vi "GenerateHeaderAndFilename.vi"(0 "Computer":string, 1 "Instrument Information":string, 2 "Test Name":string, 3 "Payload vi Name":string, 4 "Ssid":string="<tba>", 5 "Setup vi Name":string, 6 "Test Parameter File Name":string, 7 "Input Constants Keys":i32[](array[numeric]), 8 "SN":string, 9 "Input Constants Names":string[](array[string]), 10 "BenchId":string, 11 "Input Constants Values":string[](array[string])) -> (15 "Header":string[](array[string]), 18 "Filename Path":path)   [LabVIEW 2018]
uses:
  Test Result File Name Global.vi
  Automated Tests/Tetra WAM/Tetra_Globals.vi
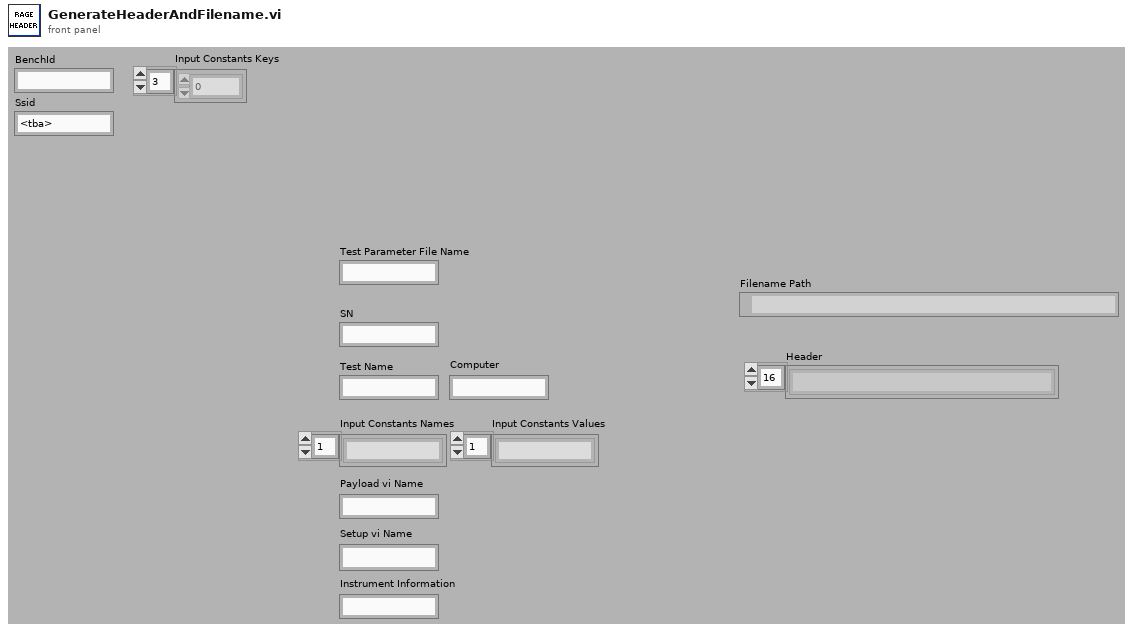
[diagram p1: front panel]
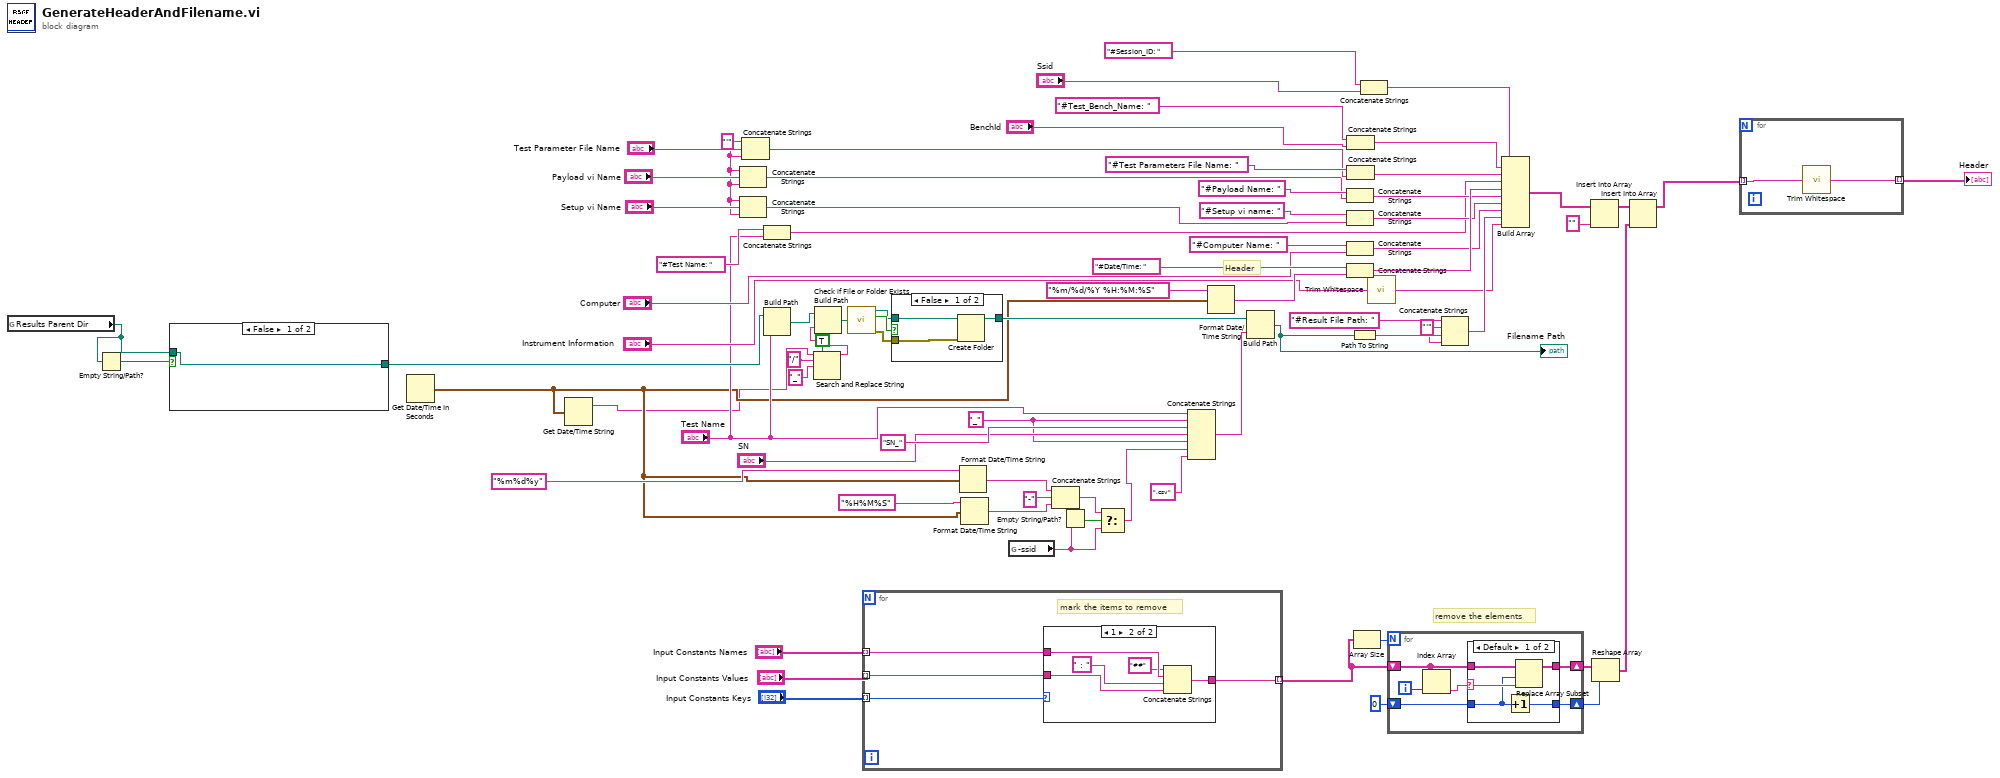
[diagram p0: block diagram]
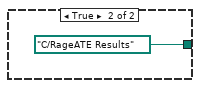
[diagram p3: hidden frame]
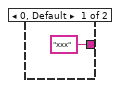
[diagram p5: hidden frame]
diagram:
  w13 = "'" ("string")
  w21 = "'" ("string")
  w36 = "_" ("string")
  # "remove the elements"
  # "Header"
  n1 = global read "Test Result File Name Global.vi" "Results Parent Dir"() -> (w33:path)
  n2 = Empty String/Path?(string/path=w33) -> (empty?=w34:bool)
  n3 = case shown="False" w34 {
    tunnel: [w80 path "C:/RageATE Results" ("base path")] -> w55
    tunnel: w33 -> [w80 _]
    frame False {
    }
    frame True {
    }
  }
  n4 = Get Date/Time In Seconds() -> (seconds since 1Jan1904=w19:timestamp)
  n5 = Get Date/Time String(seconds (now)=w19) -> (date string=w18:string)  [unwired: 2 in, 1 out]
  n6 = Concatenate Strings(w13, "Payload vi Name", w13) -> (w15:string)
  n7 = Concatenate Strings(w13, "Setup vi Name", w13) -> (w14:string)
  n8 = Concatenate Strings(w13, "Test Parameter File Name", w13) -> (w16:string)
  n9 = Concatenate Strings("#Test Name: " ("string"), "Test Name") -> (w66:string)
  n10 = Build Path(base path=w55, name or relative path="Test Name") -> (appended path=w44:path)
  n11 = Search and Replace String(replace all?=TRUE ("replace all? (F)"), input string=w18, search string="/", replace string="_" ("replace string (\"\")")) -> (result string=w43:string)  [unwired: 4 in, 3 out]
  n12 = Build Path(base path=w44, name or relative path=w43) -> (appended path=w42:path)
  n13 = call <vilib>:"Check if File or Folder Exists.vi"("path"=w42) -> ("error out"=w20:errorcluster, "file or folder exists?"=w56:bool, "dup path"=w41:path)  [unwired: 8 in]
  n14 = for {
    tunnel: "Input Constants Names" -> [w85] mode=indexing
    tunnel: "Input Constants Values" -> [w84] mode=indexing
    tunnel: [w83] -> w23 mode=indexing
    tunnel: "Input Constants Keys" -> [w82] mode=indexing
    # "mark the items to remove"
    n15 = case shown="1" w82 {
      tunnel: w85 -> [_ w91]
      tunnel: w84 -> [_ w89]
      tunnel: ["xxx" w88] -> w83
      frame 0, Default {
      }
      frame 1 {
        n16 = Concatenate Strings("##" ("string"), w91, " : " ("string"), w89) -> (w88:string)
      }
    }
  }
  n17 = case shown="False" w56 {
    tunnel: w41 -> [w94 w95]
    tunnel: [w93 w95] -> w53
    tunnel: w20 -> [w92 _]
    frame False {
      n18 = Create Folder(path (use dialog)=w94, error in=w92) -> (created path=w93:path)  [unwired: 1 in, 2 out]
    }
    frame True {
    }
  }
  n19 = Format Date/Time String(time format string (%c)="%m%d%y", seconds (now)=w19) -> (date/time string=w7:string)  [unwired: 1 in]
  n20 = Format Date/Time String(time format string (%c)="%H%M%S", seconds (now)=w19) -> (date/time string=w5:string)  [unwired: 1 in]
  n21 = global read "Tetra_Globals.vi" "-ssid"() -> (w2:string)
  n22 = Concatenate Strings(w7, "-" ("string"), w5) -> (w4:string)
  n23 = Empty String/Path?(string/path=w2) -> (empty?=w1:bool)
  n24 = Select(t=w4, s=w1, f=w2) -> (s? t:f=w3:string)
  n25 = Concatenate Strings("Test Name", w36, "SN_" ("string"), "SN", w36, w3, ".csv" ("string")) -> (w52:string)
  n26 = Format Date/Time String(time format string (%c)="%m/%d/%Y %H:%M:%S", seconds (now)=w19) -> (date/time string=w79:string)  [unwired: 1 in]
  n27 = Build Path(base path=w53, name or relative path=w52) -> (appended path=w51:path)
  "Filename Path" <- w51
  n28 = Concatenate Strings("#Payload Name: " ("string"), w15) -> (w74:string)
  n29 = Concatenate Strings("#Setup vi name: " ("string"), w14) -> (w72:string)
  n30 = Concatenate Strings("#Computer Name: " ("string"), "Computer") -> (w70:string)
  n31 = Concatenate Strings("#Date/Time: " ("string"), w79) -> (w76:string)
  n32 = Concatenate Strings("#Test_Bench_Name: " ("string"), "BenchId") -> (w30:string)
  n33 = Concatenate Strings("#Test Parameters File Name: " ("string"), w16) -> (w38:string)
  n34 = Path To String(path=w51) -> (string=w50:string)
  n35 = Array Size(array=w23) -> (size(s)=w27:i32)
  n36 = Concatenate Strings("#Session_ID: " ("string"), "Ssid") -> (w9:string)
  n37 = call <vilib>:"Trim Whitespace.vi"("string"="Instrument Information") -> ("trimmed string"=w29:string)  [unwired: 1 in]
  n38 = for {
    N: w27 -> [_]
    shift-right: [w101] -> w26
    shift-left: w23 -> [w100]
    shift-right: [w97] -> w24
    shift-left: 0 -> [w96]
    i -> [w98]
    n39 = Index Array(array=w100, index=w98) -> (element=w99:string)
    n40 = case shown="Default" w99 {
      selector: w99 -> [w104 _]
      tunnel: w100 -> [w106 w107]
      tunnel: [w105 w107] -> w101
      tunnel: [w102 w108] -> w97
      tunnel: w96 -> [w103 w108]
      frame Default {
        n41 = Increment(x=w103) -> (x+1=w102:i32)
        n42 = Replace Array Subset(array=w106, new element=w104, index=w103) -> (w105:string[])
      }
      frame "xxx" {
      }
    }
  }
  n43 = Concatenate Strings("#Result File Path: " ("string"), w21, w50, w21) -> (w57:string)
  n44 = Build Array(w9, w30, w38, w66, w76, w74, w72, w70, w57, w29) -> (w62:string[])
  n45 = Insert Into Array(array=w62, new element="" ("new element/subarray")) -> (w60:string[])  [unwired: 1 in]
  n46 = Reshape Array(w26, w24) -> (w22:string[])
  n47 = Insert Into Array(array=w60, new element=w22) -> (w12:string[])  [unwired: 1 in]
  n48 = for {
    tunnel: w12 -> [w110] mode=indexing
    tunnel: [w109] -> w11 mode=indexing
    n49 = call <vilib>:"Trim Whitespace.vi"("string"=w110) -> ("trimmed string"=w109:string)  [unwired: 1 in]
  }
  "Header" <- w11
